vi "FibrePhotometry_Ephys.vi"() -> ()   [LabVIEW 2018]
uses:
  <vilib>/DAQmx/read.llb/DAQmx Read (Analog 2D DBL NChan NSamp).vi
  <vilib>/DAQmx/write.llb/DAQmx Write (Analog 1D DBL NChan 1Samp).vi
  <vilib>/DAQmx/miscellaneous.llb/DAQmx Fill In Error Info.vi
  <vilib>/DAQmx/create/channels.llb/DAQmx Create Channel (AO-Voltage-Basic).vi
panel:
  out "Raw Data":dbl[][](graph)
  in  "Sync":bool
  in  "Amplification Factor":dbl=1.0 format="%#_13g"
  in  "Use Ephys":bool
  out "Start Time":u32
  in  "Recording":bool
  out "Recording Time":dbl
  out "Save Path":path
  out "Processed Data":dbl[][](graph)
  out "SyncPulses":waveform(dbl)[](graph)
  in  "stop":bool
  out "Loop Time":u32
  in  "Comments":string
  in  "Dir":string="C:\\Test"
  in  "Raw samples per s":dbl=2000.0 min=500.0 max=2000.0
  in  "405 LED Power":dbl=1.0 min=0.0 max=5.0
  in  "470 LED power":dbl=2.0 min=0.0 max=5.0
  in  "Frequency":dbl=10.0
  in  "Duty cycle (%)":dbl=40.0
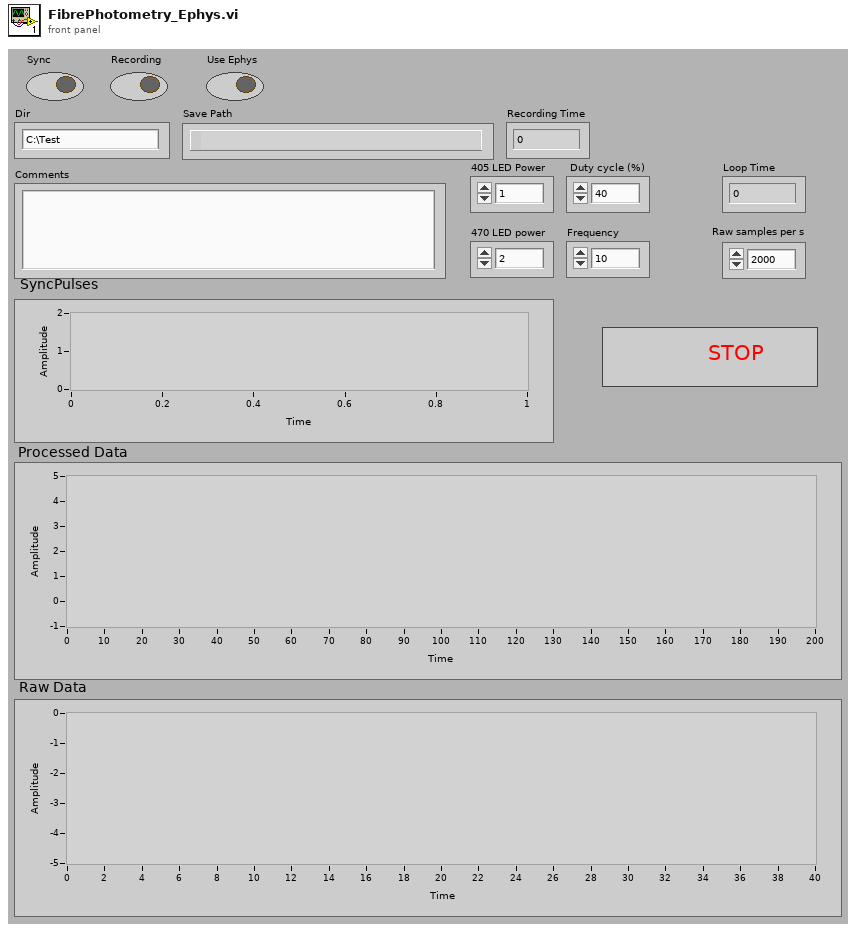
[diagram p1: front panel]
types:
  T1 = cluster{"Comments":string, "Dir":string, "Frequency":dbl, "470 LED power":dbl, "405 LED Power":dbl, "Raw samples per s":dbl, " Duty cycle (%)":dbl}
  T2 = enum16{"big-endian, network order", "native, host order", "little-endian"}
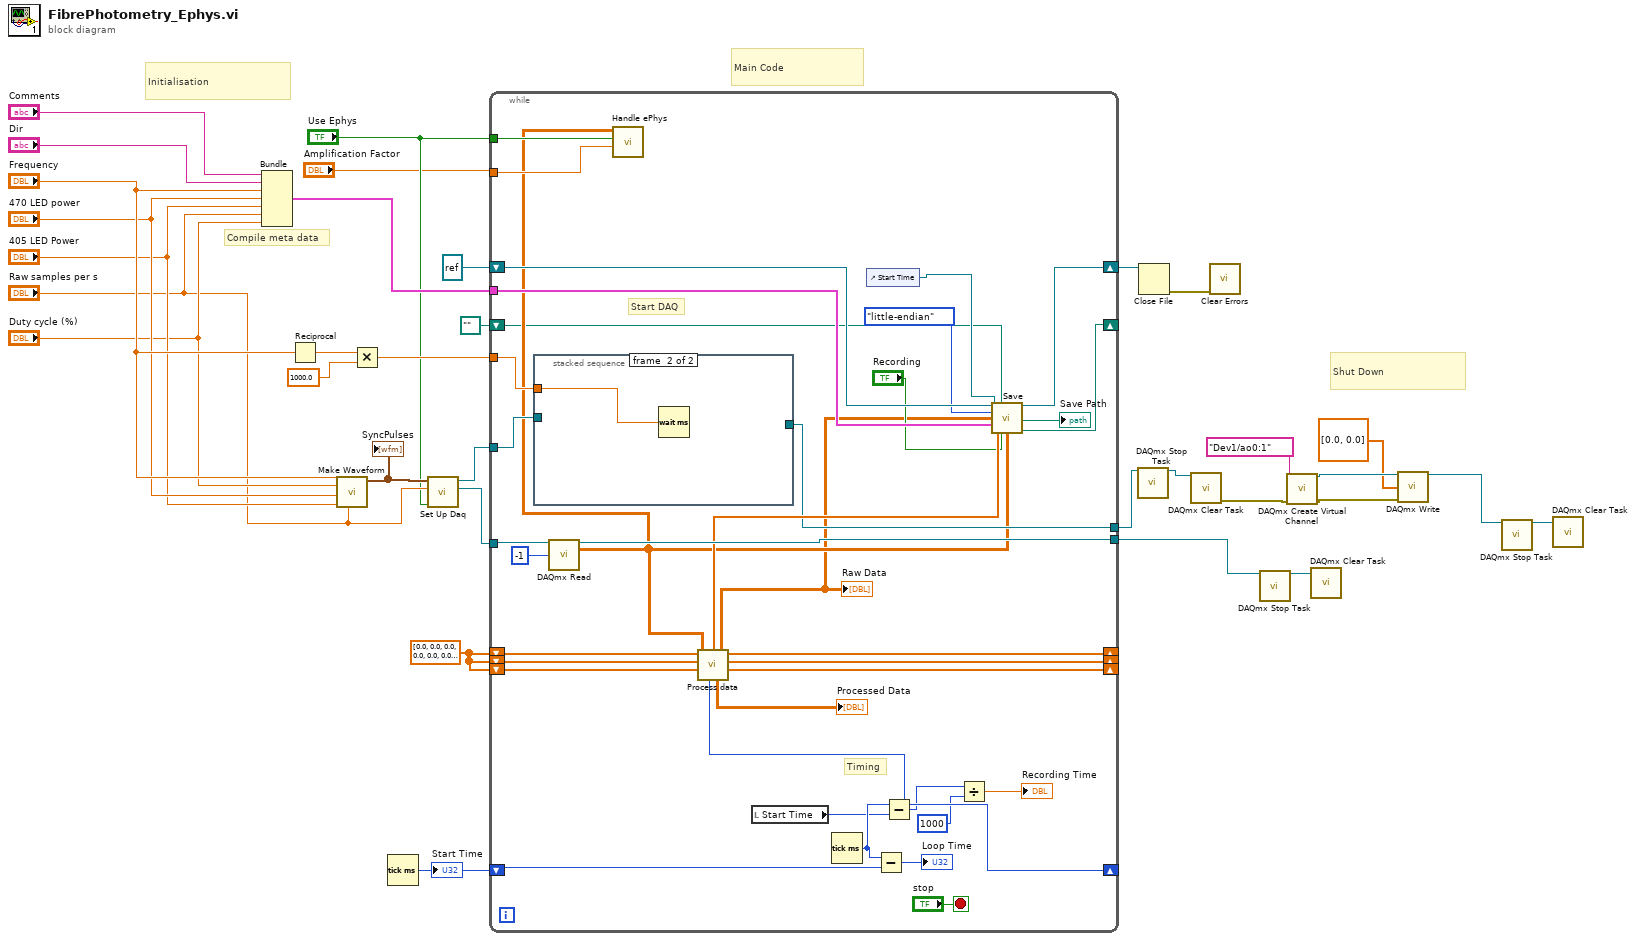
[diagram p0: block diagram]
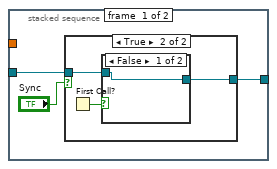
[diagram p2: hidden frame]
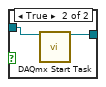
[diagram p4: hidden frame]
diagram:
  w10 = dbl[] [0.0, 0.0, 0.0, 0.0, 0.0, 0.0, 0.0, 0.0, 0.0, 0.0, 0.0, 0.0, 0.0, 0.0, 0.0, 0.0, 0.0, 0.0, 0.0, 0.0, 0.0, 0.0, 0.0, 0.0, 0.0, 0.0, 0.0, 0.0, 0.0, 0.0, 0.0, 0.0, 0.0, 0.0, 0.0, 0.0, 0.0, 0.0, 0.0, 0.0, 0.0, 0.0, 0.0, 0.0, 0.0, 0.0, 0.0, 0.0, 0.0, 0.0, 0.0, 0.0, 0.0, 0.0, 0.0, 0.0, 0.0, 0.0, 0.0, 0.0, 0.0, 0.0, 0.0, 0.0, 0.0, 0.0, 0.0, 0.0, 0.0, 0.0, 0.0, 0.0, 0.0, 0.0, 0.0, 0.0, 0.0, 0.0, 0.0, 0.0, 0.0, 0.0, 0.0, 0.0, 0.0, 0.0, 0.0, 0.0, 0.0, 0.0, 0.0, 0.0, 0.0, 0.0, 0.0, 0.0, 0.0, 0.0, 0.0, 0.0, 0.0, 0.0, 0.0, 0.0, 0.0, 0.0, 0.0, 0.0, 0.0, 0.0, 0.0, 0.0, 0.0, 0.0, 0.0, 0.0, 0.0, 0.0, 0.0, 0.0, 0.0, 0.0, 0.0, 0.0, 0.0, 0.0, 0.0, 0.0, 0.0, 0.0, 0.0, 0.0, 0.0, 0.0, 0.0, 0.0, 0.0, 0.0, 0.0, 0.0, 0.0, 0.0, 0.0, 0.0, 0.0, 0.0, 0.0, 0.0, 0.0, 0.0, 0.0, 0.0, 0.0, 0.0, 0.0, 0.0, 0.0, 0.0, 0.0, 0.0, 0.0, 0.0, 0.0, 0.0, 0.0, 0.0, 0.0, 0.0, 0.0, 0.0, 0.0, 0.0, 0.0, 0.0, 0.0, 0.0, 0.0, 0.0, 0.0, 0.0, 0.0, 0.0, 0.0, 0.0, 0.0, 0.0, 0.0, 0.0, 0.0, 0.0, 0.0, 0.0, 0.0, 0.0, 0.0, 0.0, 0.0, 0.0, 0.0, 0.0, 0.0]
  # "Shut Down"
  # "Main Code"
  # "Initialisation"
  # "Compile meta data"
  n1 = Bundle("Comments"="Comments", "Dir"="Dir", "Frequency"="Frequency", "470 LED power"="470 LED power", "405 LED Power"="405 LED Power", "Raw samples per s"="Raw samples per s", "Duty cycle (%)"="Duty cycle (%)") -> (w17:T1)  [unwired: 1 in]
  n2 = Reciprocal(x="Frequency") -> (1/x=w31:dbl)
  n3 = call "Make Waveform.vi"("Number of samples per s"="Raw samples per s", "Duty cycle (%)"="Duty cycle (%)", "405 LED Power"="405 LED Power", "470 LED power"="470 LED power", "Frequency"="Frequency") -> ("Array"=w25:waveform(dbl)[])  [unwired: 6 in]
  "SyncPulses" <- w25
  n4 = Multiply(x=w31, y=1000.0) -> (x*y=w29:dbl)
  n5 = Tick Count (ms)() -> (millisecond timer value=w27:u32)
  "Start Time" <- w27
  n6 = call "Set Up Daq.vi"("Use Ephys"="Use Ephys", "Number of samples per s"="Raw samples per s", "Array"=w25) -> ("task out 2"=w32:refnum<k21>, "Refnum out"=w33:refnum<k21>)  [unwired: 7 in]
  n7 = while {
    tunnel: w33 -> [w68]
    tunnel: w32 -> [w66]
    tunnel: w29 -> [w67]
    shift-right: [w48] -> w15
    shift-left: refnum<file> refnum ("refnum out") -> [w49]
    tunnel: [w64] -> w26
    shift-right: [w63] -> _
    shift-left: w10 -> [w62]
    shift-right: [w61] -> _
    shift-left: w10 -> [w58]
    shift-right: [w60] -> _
    shift-left: w10 -> [w59]
    shift-right: [w56] -> _
    shift-left: w27 -> [w57]
    tunnel: w17 -> [w46]
    tunnel: "Use Ephys" -> [w43]
    tunnel: "Amplification Factor" -> [w42]
    tunnel: [w41] -> w2
    shift-right: [w35] -> _
    shift-left: path "" ("new file path (Not A Path if cancelled)") -> [w34]
    stop <- "stop" stop-if-true
    # "Timing"
    # "Start DAQ"
    n8 = stacked-sequence {
      tunnel: w68 -> [w71 _]
      tunnel: [w70 _] -> w41
      tunnel: w67 -> [_ w79]
      frame #0 {
        n9 = case shown="True" "Sync" {
          tunnel: w71 -> [w72 w74]
          tunnel: [w72 w73] -> w70
          frame False {
          }
          frame True {
            n10 = First Call?() -> (First Call?: T/F=w75:bool)
            n11 = case shown="False" w75 {
              tunnel: w74 -> [w76 w78]
              tunnel: [w76 w77] -> w73
              frame False {
              }
              frame True {
                n12 = call <vilib>:"DAQmx Start Task.vi"("task/channels in"=w78) -> ("task out"=w77:refnum<k21>)  [unwired: 13 in, 1 out]
              }
            }
          }
        }
      }
      frame #1 {
        n13 = Wait (ms)(milliseconds to wait=w79) -> ()  [unwired: 1 out]
      }
    }
    n14 = call-poly <vilib>:"DAQmx Read.vi"("task/channels in"=w66, "number of samples per channel"=-1) -> ("task out"=w64:refnum<k21>, "data"=w40:dbl[][])  [unwired: 11 in, 1 out]
    n15 = call "Handle ePhys.vi"("Amplification Factor"=w42, "Use Ephys"=w43, "data"=w40) -> ()  [unwired: 9 in]
    n16 = local read "Start Time"() -> (w45:u32)
    n17 = Tick Count (ms)() -> (millisecond timer value=w56:u32)
    n18 = control-ref of="Start Time"() -> (w36:refnum<vi>)
    n19 = Subtract(x=w56, y=w57) -> (x-y=→"Loop Time":u32)
    n20 = Subtract(x=w56, y=w45) -> (x-y=w52:u32)
    n21 = call "Process data.vi"("Numeric"=w52, "data"=w40, "Array 5"=w59, "Array 4"=w58, "Array 8"=w62) -> ("Array 7"=w61:dbl[], "Array"=w39:dbl[][], "Array 9"=w63:dbl[], "Array 2"=w47:dbl[], "Array 3"=→"Processed Data":dbl[][], "Array 6"=w60:dbl[])  [unwired: 1 in]
    "Raw Data" <- w39
    n22 = Divide(x=w52, y=u32 1000) -> (x/y=→"Recording Time":dbl)
    n23 = call "Save.vi"("Digital in"=w36, "new file path (Not A Path if cancelled) in"=w34, "refnum in"=w49, "byte order (0:big-endian, network order)"=T2."little-endian", "Array"=w39, "Cluster"=w46, "Recording"="Recording", "data"=w40, "Array 2"=w47) -> ("Byte Stream File out"=w48:refnum<file>, "Save Path"=→"Save Path":path, "new file path (Not A Path if cancelled)"=w35:path)  [unwired: 4 in]
  }
  n24 = call <vilib>:"DAQmx Stop Task.vi"("task/channels in"=w2) -> ("task out"=w9:refnum<k21>)  [unwired: 13 in, 1 out]
  n25 = Close File(refnum=w15) -> (error out=w14:errorcluster)  [unwired: 1 in, 1 out]
  n26 = call <vilib>:"DAQmx Clear Task.vi"("task in"=w9) -> ("error out"=w8:errorcluster)  [unwired: 14 in]
  n27 = call <vilib>:"Clear Errors.vi"("error in (no error)"=w14) -> ()  [unwired: 5 in, 2 out]
  n28 = call <vilib>:"DAQmx Stop Task.vi"("task/channels in"=w26) -> ("task out"=w28:refnum<k21>)  [unwired: 13 in, 1 out]
  n29 = call-poly <vilib>:"DAQmx Create Virtual Channel.vi"("physical channels"=tag "Dev1/ao0:1", "error in"=w8) -> ("task out"=w5:refnum<k21>, "error out"=w6:errorcluster)  [unwired: 12 in]
  n30 = call <vilib>:"DAQmx Clear Task.vi"("task in"=w28) -> ()  [unwired: 14 in, 1 out]
  n31 = call-poly <vilib>:"DAQmx Write.vi"("task/channels in"=w5, "data"=dbl[] [0.0, 0.0], "error in"=w6) -> ("task out"=w3:refnum<k21>)  [unwired: 10 in, 2 out]
  n32 = call <vilib>:"DAQmx Stop Task.vi"("task/channels in"=w3) -> ("task out"=w24:refnum<k21>)  [unwired: 13 in, 1 out]
  n33 = call <vilib>:"DAQmx Clear Task.vi"("task in"=w24) -> ()  [unwired: 14 in, 1 out]
